vi "JoystickToSwerveCommands.vi"(9 "GyroAngle":dbl, 11 "ControllerData":T1) -> (3 "SwerveCommands":dbl[](array[numeric]))   [LabVIEW 2020]
uses:
  JoystickData.ctl
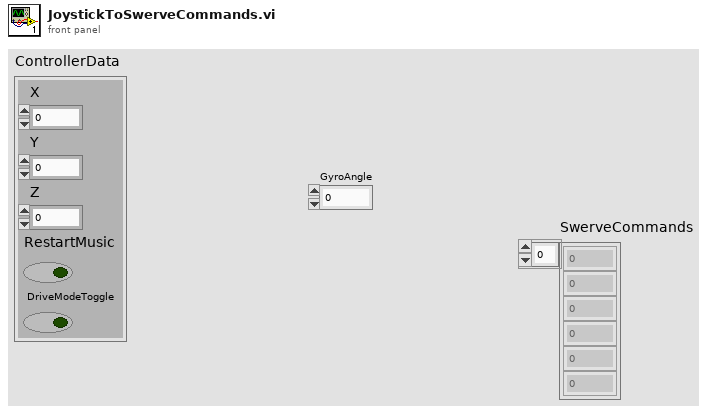
[diagram p1: front panel]
types:
  T1 = typedef "JoystickData.ctl" = cluster{"X":dbl, "Y":dbl, "Z":dbl, "RestartMusic":bool, "DriveModeToggle":bool}
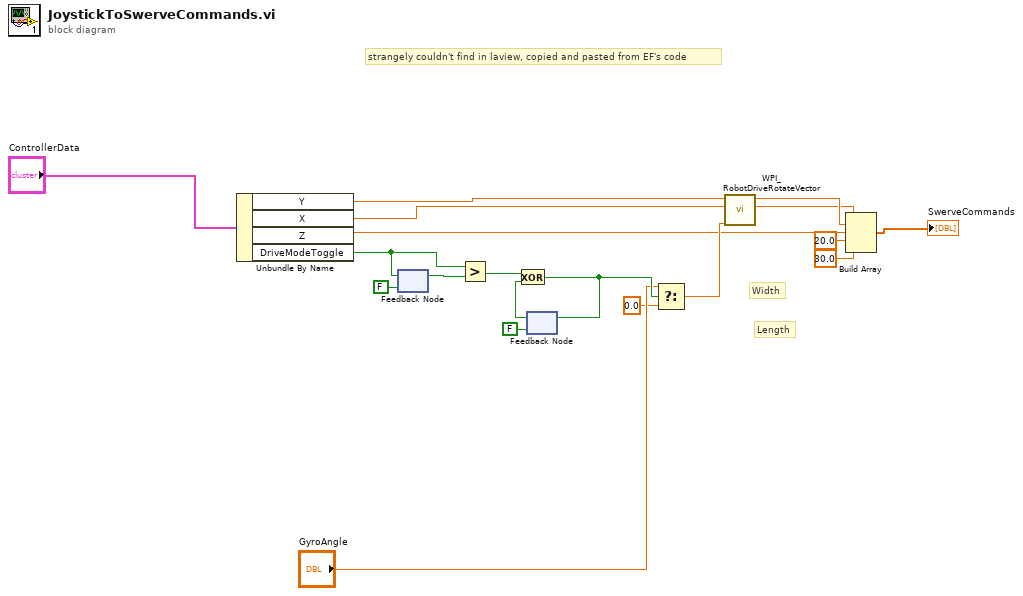
[diagram p0: block diagram]
diagram:
  # "strangely couldn't find in laview, copied and pasted from EF's code"
  # "Length"
  # "Width"
  n1 = Unbundle By Name("ControllerData") -> ("Y"=w18:dbl, "X"=w17:dbl, "Z"=w1:dbl, "DriveModeToggle"=w15:bool)
  n2 = feedback-in #1(w15) -> ()
  n3 = feedback #1(FALSE ("DriveModeToggle")) -> (w16:bool)
  n4 = Greater?(x=w15, y=w16) -> (0:w13:bool)
  n5 = feedback #2(FALSE) -> (w12:bool)
  n6 = Exclusive Or(1:w12, 2:w13) -> (0:w11:bool)
  n7 = feedback-in #2(w11) -> ()
  n8 = Select(t="GyroAngle", s=w11, f=0.0) -> (s? t:f=w7:dbl)
  n9 = call <vilib>:"WPI_RobotDriveRotateVector.vi"("Angle"=w7, "X"=w17, "Y"=w18) -> ("X'"=w2:dbl, "Y'"=w3:dbl)  [unwired: 7 out]
  n10 = Build Array(w2, w3, w1, 20.0 ("element"), 30.0 ("element")) -> (→"SwerveCommands":dbl[])
